vi "classify error.vi"(8 "error to classify":errorcluster, 10 "attempt recovery?":bool, 11 "CVT runtime in":refnum<class "CVT runtime.lvclass">) -> (0 "classified error":errorcluster, 2 "error classification":T1, 3 "CVT runtime out":refnum<class "CVT runtime.lvclass">)   [LabVIEW 2013, in "CVT runtime.lvclass"]
doc: "Allows a module to classify an error generated at any point during execution. This <b>error classification</b> can then be used by calling code to determine if execution can continue. In addition, this function can be used to allow a component to clear an error, convert an error to a warning, or attempt to recover from an error. Recovery may be attempted only if <b>attempt recovery?</b> is true."
uses:
  CVT runtime.lvclass
  <vilib>/NI/Tag Bus Module Framework/runtime/error classification.ctl
  <vilib>/NI/Tag Bus Module Framework/runtime/TBM module execution interface.lvclass
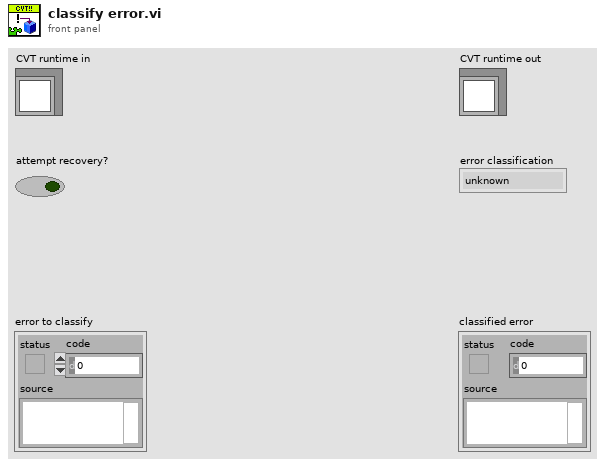
[diagram p1: front panel]
types:
  T1 = typedef "TBM module execution interface.lvclass/error classification.ctl" = enum16{"unknown", "none", "trivial", "recoverable", "critical"}
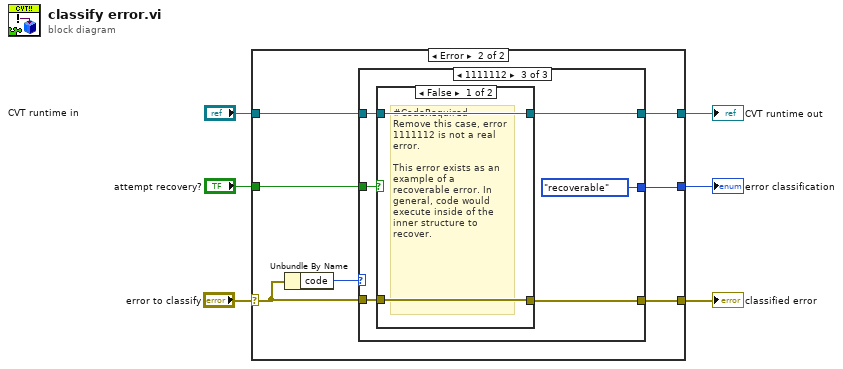
[diagram p0: block diagram]
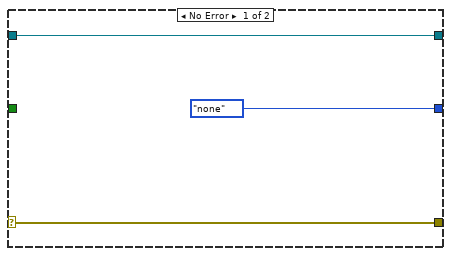
[diagram p2: hidden frame]
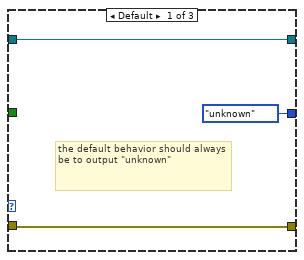
[diagram p3: hidden frame]
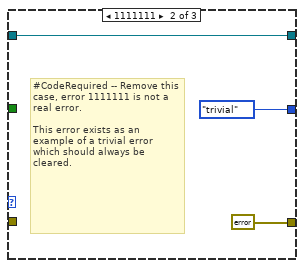
[diagram p4: hidden frame]
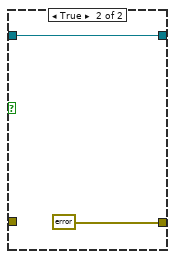
[diagram p5: hidden frame]
diagram:
  n1 = case shown="Error" "error to classify" {
    selector: "error to classify" -> [w8 w15]
    tunnel: "attempt recovery?" -> [_ w10]
    tunnel: [w9 w11] -> w4
    tunnel: "CVT runtime in" -> [w9 w12]
    tunnel: [w8 w14] -> w2
    tunnel: [error_classification."none" ("error classification") w13] -> w1
    frame No Error {
    }
    frame Error {
      n2 = Unbundle By Name(w15) -> ("code"=w16:i32)
      n3 = case shown="1111112" w16 {
        tunnel: w15 -> [w17 _ w25]
        tunnel: [w17 errorcluster {"status"=FALSE, "code"=0, "source"=""} ("error constant") w28] -> w14
        tunnel: [error_classification."unknown" ("error classification") error_classification."trivial" ("error classification") error_classification."recoverable" ("error classification")] -> w13
        tunnel: w12 -> [w18 w20 w24]
        tunnel: [w18 w20 w23] -> w11
        tunnel: w10 -> [_ _ w26]
        frame Default {
          # "the default behavior should always be to output \"unknown\""
        }
        frame 1111111 {
          # "#CodeRequired -- Remove this case, error 1111111 is not a real error.\n\nThis error exists as an example of a trivial error which should always be cleared."
        }
        frame 1111112 {
          n4 = case shown="False" w26 {
            tunnel: [w30 errorcluster {"status"=FALSE, "code"=0, "source"=""} ("error constant")] -> w28
            tunnel: w25 -> [w30 _]
            tunnel: w24 -> [w29 w31]
            tunnel: [w29 w31] -> w23
            frame False {
              # "#CodeRequired -- Remove this case, error 1111112 is not a real error.\n\nThis error exists as an example of a recoverable error. In general, code would execute inside of the inner structure to recover."
            }
            frame True {
            }
          }
        }
      }
    }
  }
  "CVT runtime out" <- w4
  "error classification" <- w1
  "classified error" <- w2
